vi "Generate Waveform.vi"(0 "signal configuration and state in":refnum<class "SV Signal.lvclass">, 5 "template waveform":waveform(dbl), 9 "samples":i32=1000, 11 "error in (no error)":errorcluster) -> (4 "signal configuration and state out":refnum<class "SV Signal.lvclass">, 6 "output waveform":waveform(dbl), 10 "samples":i32, 15 "error out":errorcluster)   [LabVIEW 2017, in "SV Signal.lvclass"]
uses:
  <vilib>/addons/_NISVFA/_Generation/Signal Generation/SV Signal/SV Signal.lvclass
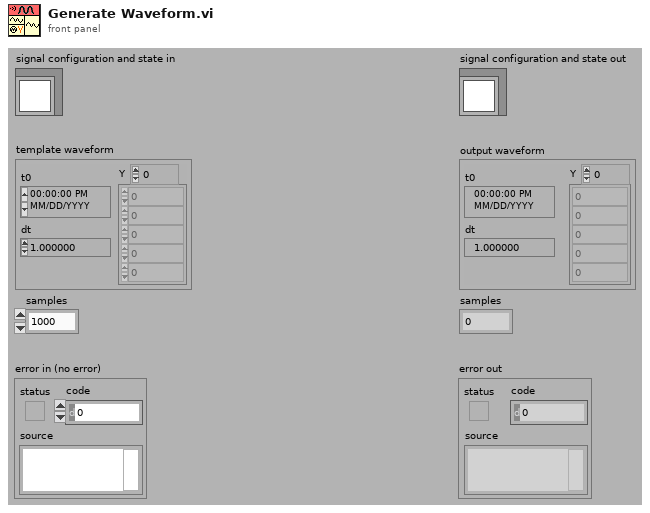
[diagram p1: front panel]
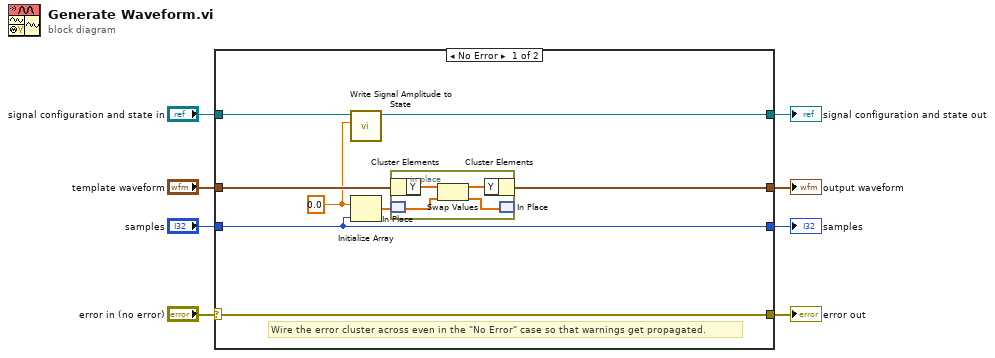
[diagram p0: block diagram]
diagram:
  n1 = case shown="No Error" "error in (no error)" {
    selector: "error in (no error)" -> [w13 w22]
    tunnel: [w13 w22] -> w7
    tunnel: [w11 w21] -> w5
    tunnel: "signal configuration and state in" -> [w12 w21]
    tunnel: [w9 _] -> w4
    tunnel: [w14 _] -> w3
    tunnel: "samples" -> [w14 _]
    tunnel: "template waveform" -> [w15 _]
    frame No Error {
      w10 = 0.0 ("element")
      # "Wire the error cluster across even in the \"No Error\" case so that warnings get propagated."
      n2 = call <vilib>:"Write Signal Amplitude to State.vi"("amplitude"=w10, "SV Signal in"=w12) -> ("SV Signal out"=w11:refnum<class "SV Signal.lvclass">)  [unwired: 8 in, 1 out]
      n3 = Initialize Array(w10, w14) -> (w16:dbl[])
      n4 = in-place {
        n5 = in-place-cluster #1(w15) -> ("Y"=w19:dbl[])
        n6 = in-place-match #2(w16) -> (w20:dbl[])
        n7 = Swap Values(12:w19, 14:w20) -> (1:w18:dbl[], 3:w17:dbl[])  [unwired: 1 in]
        n8 = in-place-cluster #1("Y"=w18) -> (w9:waveform(dbl))
        n9 = in-place-match #2(w17) -> ()  [unwired: 1 out]
      }
    }
    frame Error {
    }
  }
  "error out" <- w7
  "signal configuration and state out" <- w5
  "output waveform" <- w4
  "samples" <- w3
